vi "Write DUMMY.vi"(8 "error in (no error)":errorcluster, 10 "DUMMY":bool, 11 "Instance Handle":T1) -> (0 "error out":errorcluster, 3 "Session Handle Out":T1)   [LabVIEW 2009, in "Singleton.lvclass"]
uses:
  Singleton.lvclass
  Typedefs/Instance handle.ctl
  Singleton.lvclass/Singleton.ctl
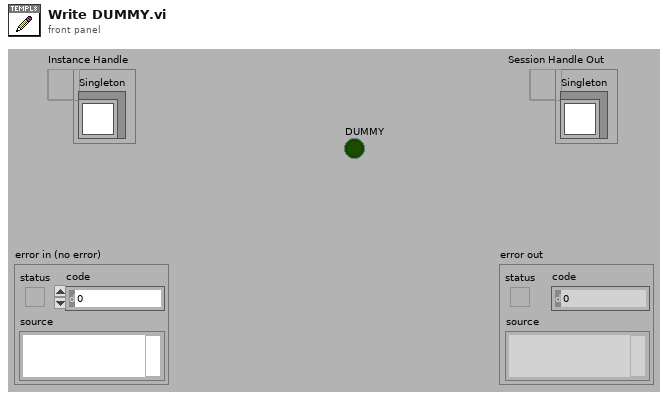
[diagram p1: front panel]
types:
  T1 = typedef "Singleton.lvclass/Instance handle.ctl" = refnum<data-value>
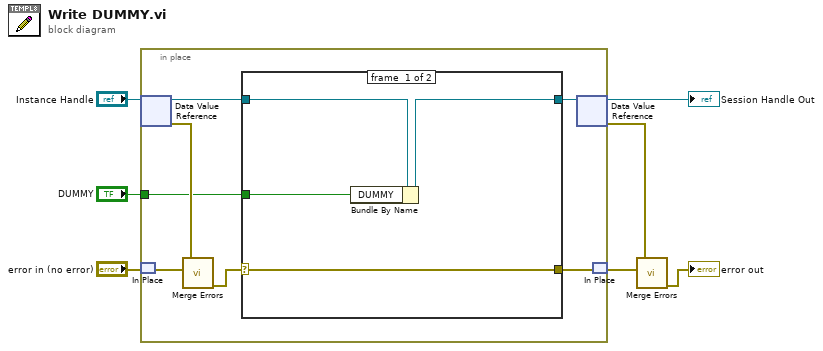
[diagram p0: block diagram]
diagram:
  n1 = in-place {
    in-place-border: "DUMMY" -> [w8]
    n2 = in-place-dvr #1("Instance Handle") -> (w10:refnum<class "Singleton.lvclass">, w11:errorcluster)
    n3 = in-place-match #2("error in (no error)") -> (w12:errorcluster)
    n4 = call <vilib>:"Merge Errors.vi"("error in 2 (no error)"=w12, "error in 1 (no error)"=w11) -> ("error out"=w14:errorcluster)  [unwired: 5 in]
    n5 = case shown="No Error" w14 {
      selector: w14 -> [w18 w19]
      tunnel: [w18 w19] -> w13
      tunnel: w10 -> [w17 w20]
      tunnel: [w16 w20] -> w9
      tunnel: w8 -> [w15 _]
      frame #0 {
        n6 = Bundle By Name(cluster=w17, "DUMMY"=w15) -> (w16:refnum<class "Singleton.lvclass">)
      }
      frame #1 {
      }
    }
    n7 = in-place-dvr #1(w9) -> (→"Session Handle Out":T1, w3:errorcluster)
    n8 = in-place-match #2(w13) -> (w2:errorcluster)
  }
  n9 = call <vilib>:"Merge Errors.vi"("error in 2 (no error)"=w2, "error in 1 (no error)"=w3) -> ("error out"=→"error out":errorcluster)  [unwired: 5 in]
